vi "VI Tree.vi"   [LabVIEW 2009, in "Keysight XSAn.lvlib"]
doc: "The VI Tree displays all the user-callable VIs of the instrument driver in an organized table."
uses:
  <instrlib>/Keysight XSAn/Keysight XSAn.lvlib
panel:
  # "XSAn"
  # "1.2.3"
  # "SEE DIAGRAM\nFOR VI Tree"
  # "© Keysight Technologies 2015-2021"
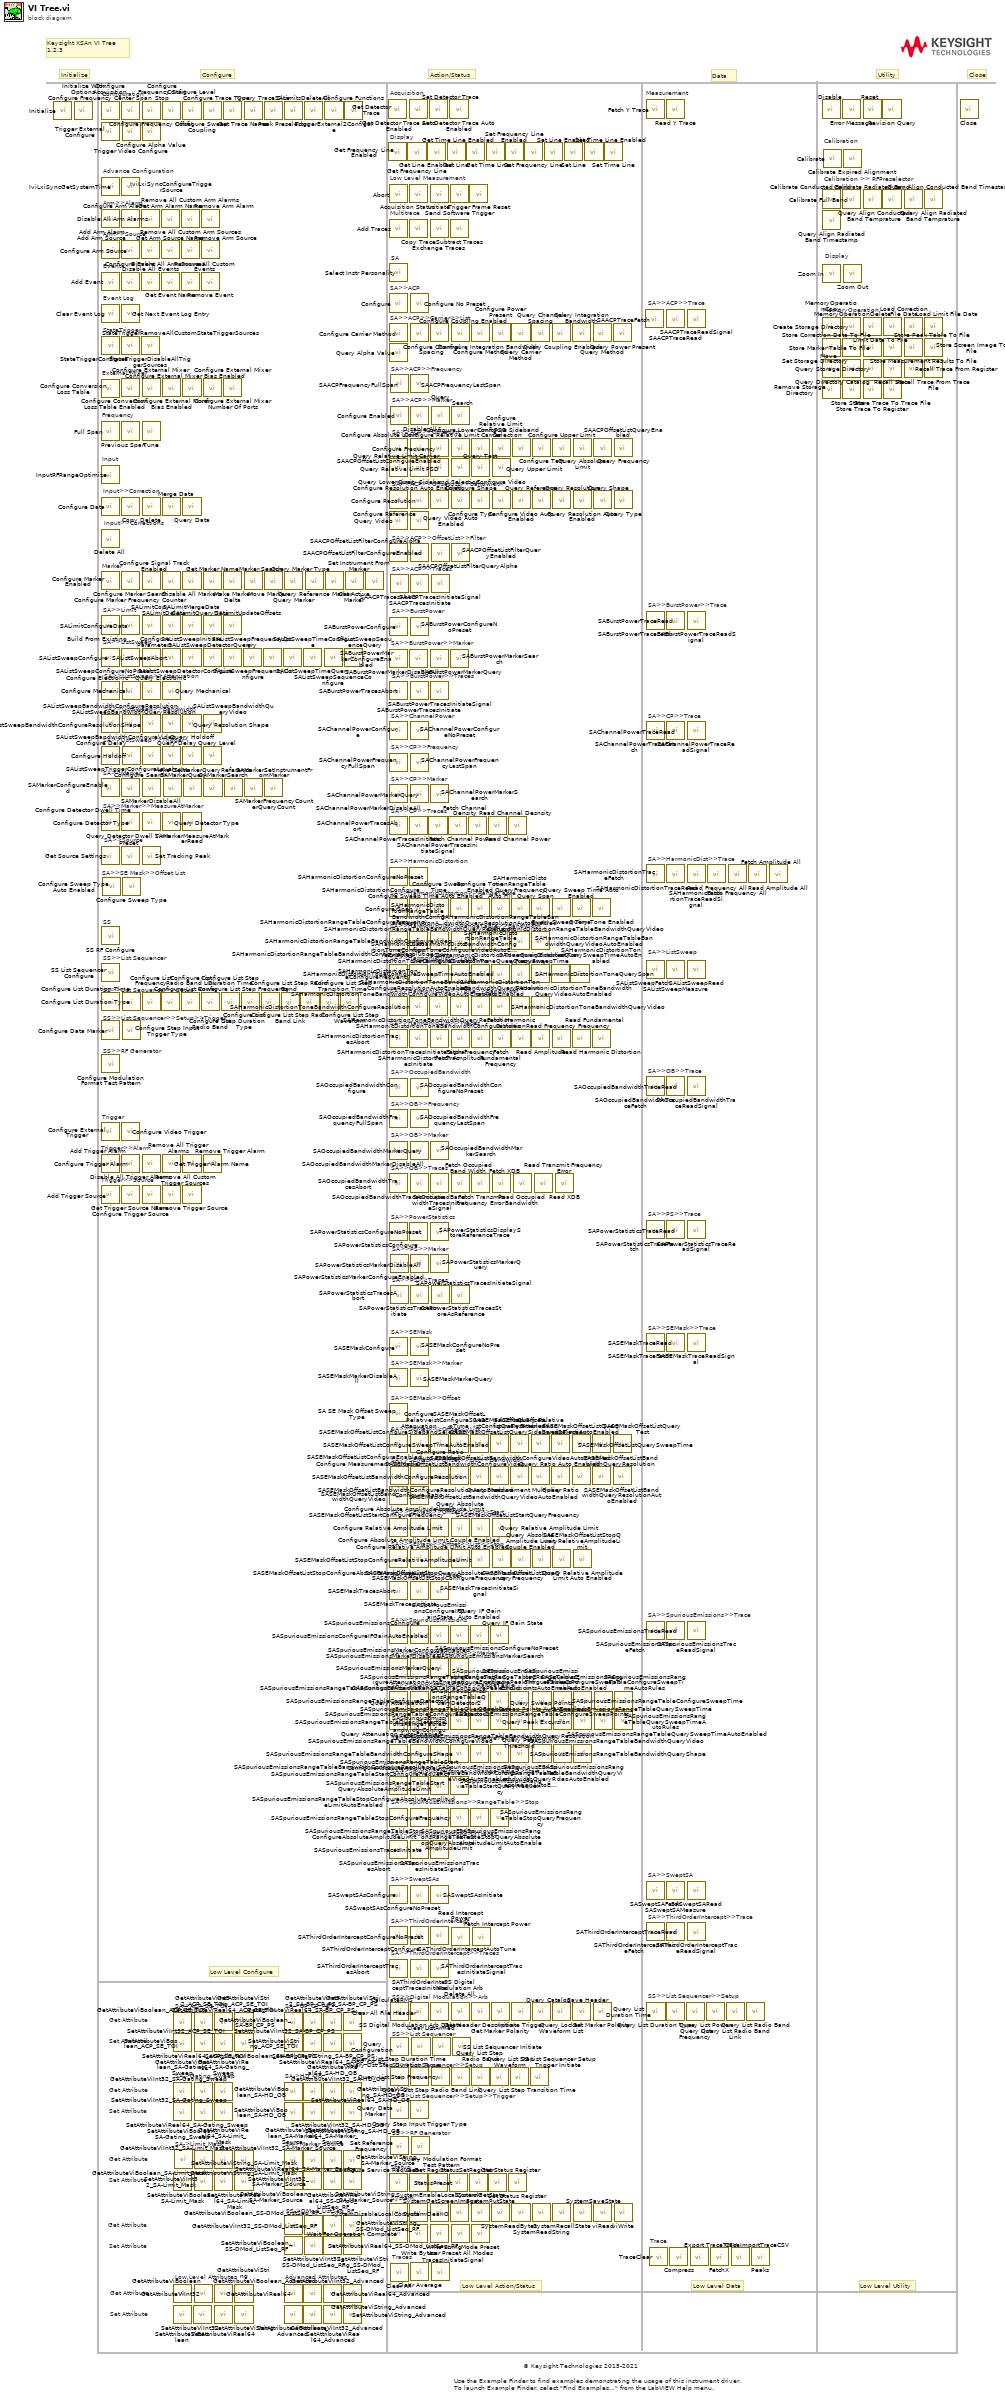
[diagram p0: block diagram]
diagram:
  # "Display"
  # "SA>>SE Mask>>Offset List"
  # "SS>>List Sequencer>>Setup"
  # "SS>>RF Generator"
  # "SS>>List Sequencer>>Setup>>Trigger"
  # "SS>>List Sequencer>>Setup"
  # "SS>>List Sequencer"
  # "SS>>RF Generator"
  # "SS>>List Sequencer>>Setup>>Trigger"
  # "SS>>List Sequencer>>Setup"
  # "SS>>List Sequencer"
  # "SS>>Digital Modulation>>Arb"
  # "SA>>SEMask>>Offset"
  # "SS->DMod_ListSeq_RF"
  # "Set Attribute"
  # "Get Attribute"
  # "SS"
  # "Advance Configuration"
  # "Set Attribute"
  # "Get Attribute"
  # "Set Attribute"
  # "Get Attribute"
  # "Set Attribute"
  # "Get Attribute"
  # "SA->HD_OB"
  # "SA->Marker_Source"
  # "SA->Limit_Mask"
  # "SA->Gating_Sweep"
  # "SA->BP_CP_PS"
  # "SA->ACP_SE_TOI"
  # "Advanced Attributes"
  # "Low Level Attributes"
  # "Trace"
  # "SA>>ListSweep"
  # "SA>>SweptSAs"
  # "SA>>SpuriousEmissions>>RangeTable>>Stop"
  # "SA>>SpuriousEmissions>>RangeTable>>Start"
  # "SA>>SpuriousEmissions>>RangeTable>>Bandwidth"
  # "SA>>SpuriousEmissions>>RangeTable"
  # "SA>>SpuriousEmissions"
  # "SA>>SEMask>>Offset>>List>>Stop"
  # "SA>>SEMask>>Offset>>List>>Start"
  # "SA>>SEMask>>Offset>>List>>Bandwidth"
  # "SA>>SEMask>>Offset>>List"
  # "SA>>Marker>>MeasureAtMarker"
  # "SA>>Marker"
  # "SA>>ListSweep>>Trigger"
  # "SA>>ListSweep>>Bandwidth"
  # "SA>>ListSweep>>Attenuation"
  # "SA>>ListSweep"
  # "SA>>HarmonicDist>>Tone>>Bandwidth"
  # "SA>>HarmonicDist>>Tone"
  # "SA>>HarmonicDist>>RangeTable>>Bandwidth"
  # "SA>>HarmonicDistortion>>RangeTable"
  # "SA>>ACP>>OffsetList>>Filter"
  # "SA>>ACP>>OffsetList>>Bandwidth"
  # "SA>>ACP>>OffsetList"
  # "Set Attribute"
  # "Get Attribute"
  # "© Keysight Technologies 2015-2021"
  # "Low Level Utility"
  # "Low Level Configure"
  # "Low Level Action/Status"
  # "Low Level Data"
  # "Action/Status"
  # "Keysight XSAn VI Tree\n1.2.3"
  # "Close"
  # "Utility"
  # "Data"
  # "Configure"
  # "Initialize"
  # "Use the Example Finder to find examples demonstrating the usage of this instrument driver.\nTo launch Example Finder, select \"Find Examples...\" from the LabVIEW Help menu."
  # "Traces"
  # "System"
  # "Status"
  # "StateTrigger"
  # "SA>>ThirdOrderIntercept>>Traces"
  # "SA>>ThirdOrderIntercept>>Trace"
  # "SA>>ThirdOrderIntercept"
  # "SA>>SweptSA"
  # "SA>>SpuriousEmissions>>Traces"
  # "SA>>SpuriousEmissions>>Trace"
  # "SA>>SpuriousEmissions>>Marker"
  # "SA>>Source"
  # "SA>>SEMask>>Traces"
  # "SA>>SEMask>>Trace"
  # "SA>>SEMask>>Marker"
  # "SA>>SEMask"
  # "SA>>PS>>Traces"
  # "SA>>PS>>Trace"
  # "SA>>PS>>Marker"
  # "SA>>PowerStatistics"
  # "SA>>OB>>Traces"
  # "SA>>OB>>Trace"
  # "SA>>OB>>Marker"
  # "SA>>OB>>Frequency"
  # "SA>>OccupiedBandwidth"
  # "SA>>Limit"
  # "SA>>HarmonicDist>>Traces"
  # "SA>>HarmonicDist>>Trace"
  # "SA>>HarmonicDistortion"
  # "SA>>CP>>Traces"
  # "SA>>CP>>Trace"
  # "SA>>CP>>Marker"
  # "SA>>CP>>Frequency"
  # "SA>>ChannelPower"
  # "SA>>BurstPower>>Traces"
  # "SA>>BurstPower>>Trace"
  # "SA>>BurstPower>>Marker"
  # "SA>>BurstPower"
  # "SA>>ACP>>Traces"
  # "SA>>ACP>>Trace"
  # "SA>>ACP>>Marker"
  # "SA>>ACP>>Frequency"
  # "SA>>ACP>>Carrier>>List"
  # "SA>>ACP"
  # "SA"
  # "MemoryOperation"
  # "Low Level Measurement"
  # "Measurement"
  # "Input>>Corrections"
  # "Input>>Correction"
  # "Input"
  # "Frequency"
  # "Event Log"
  # "Display"
  # "Trigger>>Source"
  # "Trigger>>Alarm"
  # "Trigger"
  # "Multitrace"
  # "Marker"
  # "External Mixer"
  # "Event"
  # "Arm>>Source"
  # "Arm>>Alarm"
  # "Configuration"
  # "Calibration >> RFPreselector"
  # "Calibration"
  # "Acquisition"
  n1 = call <instrlib>:"Initialize.vi"() -> ()  [unwired: 10 in, 2 out]
  n2 = call <instrlib>:"Initialize With Options.vi"() -> ()  [unwired: 10 in, 2 out]
  n3 = call <instrlib>:"Configure Acquisition.vi"() -> ()  [unwired: 10 in, 2 out]
  n4 = call <instrlib>:"Trigger External Configure.vi"() -> ()  [unwired: 10 in, 2 out]
  n5 = call <instrlib>:"Configure Conversion Loss Table.vi"() -> ()  [unwired: 10 in, 2 out]
  n6 = call <instrlib>:"Full Span.vi"() -> ()  [unwired: 10 in, 2 out]
  n7 = call <instrlib>:"InputRFRangeOptimize.vi"() -> ()  [unwired: 10 in, 2 out]
  n8 = call <instrlib>:"Configure Data.vi"() -> ()  [unwired: 10 in, 2 out]
  n9 = call <instrlib>:"Delete All.vi"() -> ()  [unwired: 10 in, 2 out]
  n10 = call <instrlib>:"Configure Marker Enabled.vi"() -> ()  [unwired: 10 in, 2 out]
  n11 = call <instrlib>:"Build From Existing.vi"() -> ()  [unwired: 10 in, 2 out]
  n12 = call <instrlib>:"SAListSweepConfigure.vi"() -> ()  [unwired: 10 in, 2 out]
  n13 = call <instrlib>:"SAMarkerConfigureEnabled.vi"() -> ()  [unwired: 10 in, 2 out]
  n14 = call <instrlib>:"Configure Detector Dwell Time.vi"() -> ()  [unwired: 10 in, 2 out]
  n15 = call <instrlib>:"Get Source Settings.vi"() -> ()  [unwired: 8 in, 4 out]
  n16 = call <instrlib>:"Configure External Trigger.vi"() -> ()  [unwired: 10 in, 2 out]
  n17 = call <instrlib>:"Add Trigger Alarm.vi"() -> ()  [unwired: 10 in, 2 out]
  n18 = call <instrlib>:"Add Trigger Source.vi"() -> ()  [unwired: 10 in, 2 out]
  n19 = call <instrlib>:"IviLxiSyncGetSystemTime.vi"() -> ()  [unwired: 8 in, 4 out]
  n20 = call <instrlib>:"Add Arm Alarm.vi"() -> ()  [unwired: 10 in, 2 out]
  n21 = call <instrlib>:"Add Arm Source.vi"() -> ()  [unwired: 10 in, 2 out]
  n22 = call <instrlib>:"Add Event.vi"() -> ()  [unwired: 10 in, 2 out]
  n23 = call <instrlib>:"Clear Event Log.vi"() -> ()  [unwired: 10 in, 2 out]
  n24 = call <instrlib>:"StateTriggerConfigure.vi"() -> ()  [unwired: 10 in, 2 out]
  n25 = call <instrlib>:"Configure Electronic.vi"() -> ()  [unwired: 10 in, 2 out]
  n26 = call <instrlib>:"SAListSweepBandwidthConfigureResolution.vi"() -> ()  [unwired: 10 in, 2 out]
  n27 = call <instrlib>:"Configure Delay.vi"() -> ()  [unwired: 10 in, 2 out]
  n28 = call <instrlib>:"SS RF Configure.vi"() -> ()  [unwired: 10 in, 2 out]
  n29 = call <instrlib>:"SS List Sequencer Configure.vi"() -> ()  [unwired: 14 in, 2 out]
  n30 = call <instrlib>:"Configure List Duration Time.vi"() -> ()  [unwired: 10 in, 2 out]
  n31 = call <instrlib>:"Configure Data Marker.vi"() -> ()  [unwired: 10 in, 2 out]
  n32 = call <instrlib>:"Configure Modulation Format Test Pattern.vi"() -> ()  [unwired: 10 in, 2 out]
  n33 = call <instrlib>:"Configure Sweep Type Auto Enabled.vi"() -> ()  [unwired: 10 in, 2 out]
  n34 = call <instrlib>:"Configure Frequency Center Span.vi"() -> ()  [unwired: 10 in, 2 out]
  n35 = call <instrlib>:"IviLxiSyncConfigureTriggerSource.vi"() -> ()  [unwired: 10 in, 2 out]
  n36 = call <instrlib>:"Configure Arm Alarm.vi"() -> ()  [unwired: 10 in, 2 out]
  n37 = call <instrlib>:"Configure Arm Source.vi"() -> ()  [unwired: 10 in, 2 out]
  n38 = call <instrlib>:"Configure Event.vi"() -> ()  [unwired: 10 in, 2 out]
  n39 = call <instrlib>:"Get Next Event Log Entry.vi"() -> ()  [unwired: 9 in, 3 out]
  n40 = call <instrlib>:"StateTriggerRemoveAllCustomStateTriggerSources.vi"() -> ()  [unwired: 10 in, 2 out]
  n41 = call <instrlib>:"Configure Conversion Loss Table Enabled.vi"() -> ()  [unwired: 10 in, 2 out]
  n42 = call <instrlib>:"Previous Span.vi"() -> ()  [unwired: 10 in, 2 out]
  n43 = call <instrlib>:"Copy.vi"() -> ()  [unwired: 10 in, 2 out]
  n44 = call <instrlib>:"Configure Marker Frequency Counter.vi"() -> ()  [unwired: 10 in, 2 out]
  n45 = call <instrlib>:"SALimitConfigureData.vi"() -> ()  [unwired: 10 in, 2 out]
  n46 = call <instrlib>:"SAListSweepConfigureNoPreset.vi"() -> ()  [unwired: 10 in, 2 out]
  n47 = call <instrlib>:"Configure Search.vi"() -> ()  [unwired: 10 in, 2 out]
  n48 = call <instrlib>:"Configure Detector Type.vi"() -> ()  [unwired: 10 in, 2 out]
  n49 = call <instrlib>:"Preset.vi"() -> ()  [unwired: 10 in, 2 out]
  n50 = call <instrlib>:"Configure Video Trigger.vi"() -> ()  [unwired: 10 in, 2 out]
  n51 = call <instrlib>:"Configure Trigger Alarm.vi"() -> ()  [unwired: 10 in, 2 out]
  n52 = call <instrlib>:"Configure Trigger Source.vi"() -> ()  [unwired: 10 in, 2 out]
  n53 = call <instrlib>:"Trigger Video Configure.vi"() -> ()  [unwired: 10 in, 2 out]
  n54 = call <instrlib>:"Configure Mechanical.vi"() -> ()  [unwired: 10 in, 2 out]
  n55 = call <instrlib>:"SAListSweepBandwidthConfigureResolutionShape.vi"() -> ()  [unwired: 10 in, 2 out]
  n56 = call <instrlib>:"Configure Holdoff.vi"() -> ()  [unwired: 10 in, 2 out]
  n57 = call <instrlib>:"Configure List Duration Type.vi"() -> ()  [unwired: 10 in, 2 out]
  n58 = call <instrlib>:"Configure Step Input Trigger Type.vi"() -> ()  [unwired: 10 in, 2 out]
  n59 = call <instrlib>:"Configure Sweep Type.vi"() -> ()  [unwired: 10 in, 2 out]
  n60 = call <instrlib>:"Disable All Arm Alarms.vi"() -> ()  [unwired: 10 in, 2 out]
  n61 = call <instrlib>:"Disable All Arm Sources.vi"() -> ()  [unwired: 10 in, 2 out]
  n62 = call <instrlib>:"Disable All Events.vi"() -> ()  [unwired: 10 in, 2 out]
  n63 = call <instrlib>:"StateTriggerDisableAllTriggerSources.vi"() -> ()  [unwired: 10 in, 2 out]
  n64 = call <instrlib>:"Configure Frequency Offset.vi"() -> ()  [unwired: 10 in, 2 out]
  n65 = call <instrlib>:"Configure Alpha Value.vi"() -> ()  [unwired: 10 in, 2 out]
  n66 = call <instrlib>:"Configure External Mixer.vi"() -> ()  [unwired: 10 in, 2 out]
  n67 = call <instrlib>:"Tune.vi"() -> ()  [unwired: 10 in, 2 out]
  n68 = call <instrlib>:"Delete.vi"() -> ()  [unwired: 10 in, 2 out]
  n69 = call <instrlib>:"Configure Marker Search.vi"() -> ()  [unwired: 10 in, 2 out]
  n70 = call <instrlib>:"SALimitCopy.vi"() -> ()  [unwired: 10 in, 2 out]
  n71 = call <instrlib>:"Configure Parameters.vi"() -> ()  [unwired: 14 in, 2 out]
  n72 = call <instrlib>:"Query Electronic.vi"() -> ()  [unwired: 8 in, 4 out]
  n73 = call <instrlib>:"Query Detector Dwell Time.vi"() -> ()  [unwired: 9 in, 3 out]
  n74 = call <instrlib>:"Set Tracking Peak.vi"() -> ()  [unwired: 10 in, 2 out]
  n75 = call <instrlib>:"Configure List Frequency.vi"() -> ()  [unwired: 10 in, 2 out]
  n76 = call <instrlib>:"Disable All Trigger Alarms.vi"() -> ()  [unwired: 10 in, 2 out]
  n77 = call <instrlib>:"Get Trigger Source Name.vi"() -> ()  [unwired: 9 in, 3 out]
  n78 = call <instrlib>:"SAListSweepBandwidthConfigureVideo.vi"() -> ()  [unwired: 10 in, 2 out]
  n79 = call <instrlib>:"SAListSweepTriggerConfigureLevel.vi"() -> ()  [unwired: 10 in, 2 out]
  n80 = call <instrlib>:"SAMarkerDisableAll.vi"() -> ()  [unwired: 10 in, 2 out]
  n81 = call <instrlib>:"Get Arm Alarm Name.vi"() -> ()  [unwired: 9 in, 3 out]
  n82 = call <instrlib>:"Get Arm Source Name.vi"() -> ()  [unwired: 9 in, 3 out]
  n83 = call <instrlib>:"Get Event Name.vi"() -> ()  [unwired: 9 in, 3 out]
  n84 = call <instrlib>:"Configure List Power.vi"() -> ()  [unwired: 10 in, 2 out]
  n85 = call <instrlib>:"Configure Frequency Start Stop.vi"() -> ()  [unwired: 10 in, 2 out]
  n86 = call <instrlib>:"Configure External Mixer Bias.vi"() -> ()  [unwired: 10 in, 2 out]
  n87 = call <instrlib>:"Merge Data.vi"() -> ()  [unwired: 10 in, 2 out]
  n88 = call <instrlib>:"Configure Signal Track Enabled.vi"() -> ()  [unwired: 10 in, 2 out]
  n89 = call <instrlib>:"SALimitDelete.vi"() -> ()  [unwired: 10 in, 2 out]
  n90 = call <instrlib>:"SAListSweepAbort.vi"() -> ()  [unwired: 10 in, 2 out]
  n91 = call <instrlib>:"Query Mechanical.vi"() -> ()  [unwired: 8 in, 4 out]
  n92 = call <instrlib>:"SAListSweepBandwidthQueryResolution.vi"() -> ()  [unwired: 8 in, 4 out]
  n93 = call <instrlib>:"Query Delay.vi"() -> ()  [unwired: 8 in, 4 out]
  n94 = call <instrlib>:"Query Detector Type.vi"() -> ()  [unwired: 9 in, 3 out]
  n95 = call <instrlib>:"Get Trigger Alarm Name.vi"() -> ()  [unwired: 9 in, 3 out]
  n96 = call <instrlib>:"Remove All Custom Trigger Sources.vi"() -> ()  [unwired: 10 in, 2 out]
  n97 = call <instrlib>:"Make Delta.vi"() -> ()  [unwired: 10 in, 2 out]
  n98 = call <instrlib>:"GetAttributeViBoolean_ACP_SE_TOI.vi"() -> ()  [unwired: 9 in, 3 out]
  n99 = call <instrlib>:"SetAttributeViBoolean_ACP_SE_TOI.vi"() -> ()  [unwired: 10 in, 2 out]
  n100 = call <instrlib>:"GetAttributeViBoolean_SA-Gating_Sweep.vi"() -> ()  [unwired: 9 in, 3 out]
  n101 = call <instrlib>:"SetAttributeViBoolean_SA-Gating_Sweep.vi"() -> ()  [unwired: 10 in, 2 out]
  n102 = call <instrlib>:"SetAttributeViBoolean_SA-Limit_Mask.vi"() -> ()  [unwired: 10 in, 2 out]
  n103 = call <instrlib>:"GetAttributeViBoolean.vi"() -> ()  [unwired: 9 in, 3 out]
  n104 = call <instrlib>:"SetAttributeViBoolean.vi"() -> ()  [unwired: 10 in, 2 out]
  n105 = call <instrlib>:"GetAttributeViBoolean_SA-Limit_Mask.vi"() -> ()  [unwired: 9 in, 3 out]
  n106 = call <instrlib>:"Remove All Custom Arm Alarms.vi"() -> ()  [unwired: 10 in, 2 out]
  n107 = call <instrlib>:"Remove All Custom Arm Sources.vi"() -> ()  [unwired: 10 in, 2 out]
  n108 = call <instrlib>:"Remove All Custom Events.vi"() -> ()  [unwired: 10 in, 2 out]
  n109 = call <instrlib>:"Configure List Radio Band Link.vi"() -> ()  [unwired: 10 in, 2 out]
  n110 = call <instrlib>:"Configure Level.vi"() -> ()  [unwired: 10 in, 2 out]
  n111 = call <instrlib>:"Configure External Mixer Bias Enabled.vi"() -> ()  [unwired: 10 in, 2 out]
  n112 = call <instrlib>:"Query Data.vi"() -> ()  [unwired: 8 in, 4 out]
  n113 = call <instrlib>:"Disable All Markers.vi"() -> ()  [unwired: 10 in, 2 out]
  n114 = call <instrlib>:"SALimitMergeData.vi"() -> ()  [unwired: 10 in, 2 out]
  n115 = call <instrlib>:"SAListSweepInitiate.vi"() -> ()  [unwired: 10 in, 2 out]
  n116 = call <instrlib>:"Query Resolution Shape.vi"() -> ()  [unwired: 8 in, 4 out]
  n117 = call <instrlib>:"Query Holdoff.vi"() -> ()  [unwired: 8 in, 4 out]
  n118 = call <instrlib>:"SAMarkerMeasureAtMarkerRead.vi"() -> ()  [unwired: 8 in, 4 out]
  n119 = call <instrlib>:"Remove All Trigger Alarms.vi"() -> ()  [unwired: 10 in, 2 out]
  n120 = call <instrlib>:"Remove Trigger Source.vi"() -> ()  [unwired: 10 in, 2 out]
  n121 = call <instrlib>:"SAMarkerQuery.vi"() -> ()  [unwired: 8 in, 4 out]
  n122 = call <instrlib>:"SetAttributeViInt32.vi"() -> ()  [unwired: 10 in, 2 out]
  n123 = call <instrlib>:"GetAttributeViInt32_ACP_SE_TOI.vi"() -> ()  [unwired: 9 in, 3 out]
  n124 = call <instrlib>:"SetAttributeViInt32_ACP_SE_TOI.vi"() -> ()  [unwired: 10 in, 2 out]
  n125 = call <instrlib>:"GetAttributeViInt32_SA-Gating_Sweep.vi"() -> ()  [unwired: 9 in, 3 out]
  n126 = call <instrlib>:"SetAttributeViInt32_SA-Gating_Sweep.vi"() -> ()  [unwired: 10 in, 2 out]
  n127 = call <instrlib>:"GetAttributeViInt32_SA-Limit_Mask.vi"() -> ()  [unwired: 9 in, 3 out]
  n128 = call <instrlib>:"SetAttributeViInt32_SA-Limit_Mask.vi"() -> ()  [unwired: 10 in, 2 out]
  n129 = call <instrlib>:"GetAttributeViInt32.vi"() -> ()  [unwired: 9 in, 3 out]
  n130 = call <instrlib>:"Remove Arm Alarm.vi"() -> ()  [unwired: 10 in, 2 out]
  n131 = call <instrlib>:"Remove Arm Source.vi"() -> ()  [unwired: 10 in, 2 out]
  n132 = call <instrlib>:"Remove Event.vi"() -> ()  [unwired: 10 in, 2 out]
  n133 = call <instrlib>:"Configure List Radio Band.vi"() -> ()  [unwired: 10 in, 2 out]
  n134 = call <instrlib>:"Configure Sweep Coupling.vi"() -> ()  [unwired: 10 in, 2 out]
  n135 = call <instrlib>:"Configure External Mixer Enabled.vi"() -> ()  [unwired: 10 in, 2 out]
  n136 = call <instrlib>:"Get Marker Name.vi"() -> ()  [unwired: 9 in, 3 out]
  n137 = call <instrlib>:"SALimitQueryData.vi"() -> ()  [unwired: 8 in, 4 out]
  n138 = call <instrlib>:"SAListSweepDetectorConfigure.vi"() -> ()  [unwired: 10 in, 2 out]
  n139 = call <instrlib>:"SAListSweepBandwidthQueryVideo.vi"() -> ()  [unwired: 8 in, 4 out]
  n140 = call <instrlib>:"Query Level.vi"() -> ()  [unwired: 8 in, 4 out]
  n141 = call <instrlib>:"Remove Trigger Alarm.vi"() -> ()  [unwired: 10 in, 2 out]
  n142 = call <instrlib>:"SAMarkerQueryReference.vi"() -> ()  [unwired: 8 in, 4 out]
  n143 = call <instrlib>:"GetAttributeViReal64_ACP_SE_TOI.vi"() -> ()  [unwired: 9 in, 3 out]
  n144 = call <instrlib>:"SetAttributeViReal64_ACP_SE_TOI.vi"() -> ()  [unwired: 10 in, 2 out]
  n145 = call <instrlib>:"GetAttributeViReal64_SA-Gating_Sweep.vi"() -> ()  [unwired: 9 in, 3 out]
  n146 = call <instrlib>:"SetAttributeViReal64_SA-Gating_Sweep.vi"() -> ()  [unwired: 10 in, 2 out]
  n147 = call <instrlib>:"GetAttributeViReal64_SA-Limit_Mask.vi"() -> ()  [unwired: 9 in, 3 out]
  n148 = call <instrlib>:"SetAttributeViReal64_SA-Limit_Mask.vi"() -> ()  [unwired: 10 in, 2 out]
  n149 = call <instrlib>:"GetAttributeViReal64.vi"() -> ()  [unwired: 9 in, 3 out]
  n150 = call <instrlib>:"SetAttributeViReal64.vi"() -> ()  [unwired: 10 in, 2 out]
  n151 = call <instrlib>:"Configure List Step Duration Time.vi"() -> ()  [unwired: 10 in, 2 out]
  n152 = call <instrlib>:"Configure Trace Type.vi"() -> ()  [unwired: 10 in, 2 out]
  n153 = call <instrlib>:"Configure External Mixer Number Of Ports.vi"() -> ()  [unwired: 10 in, 2 out]
  n154 = call <instrlib>:"Make Marker Delta.vi"() -> ()  [unwired: 10 in, 2 out]
  n155 = call <instrlib>:"SALimitUpdateOffsets.vi"() -> ()  [unwired: 10 in, 2 out]
  n156 = call <instrlib>:"SAListSweepDetectorQuery.vi"() -> ()  [unwired: 8 in, 4 out]
  n157 = call <instrlib>:"SAMarkerSearch.vi"() -> ()  [unwired: 10 in, 2 out]
  n158 = call <instrlib>:"GetAttributeViString_ACP_SE_TOI.vi"() -> ()  [unwired: 9 in, 3 out]
  n159 = call <instrlib>:"SetAttributeViString_ACP_SE_TOI.vi"() -> ()  [unwired: 10 in, 2 out]
  n160 = call <instrlib>:"GetAttributeViString_SA-Limit_Mask.vi"() -> ()  [unwired: 9 in, 3 out]
  n161 = call <instrlib>:"SetAttributeViString_SA-Limit_Mask.vi"() -> ()  [unwired: 10 in, 2 out]
  n162 = call <instrlib>:"GetAttributeViString.vi"() -> ()  [unwired: 9 in, 3 out]
  n163 = call <instrlib>:"SetAttributeViString.vi"() -> ()  [unwired: 10 in, 2 out]
  n164 = call <instrlib>:"Configure List Step Duration Type.vi"() -> ()  [unwired: 10 in, 2 out]
  n165 = call <instrlib>:"SAListSweepFrequencyConfigure.vi"() -> ()  [unwired: 10 in, 2 out]
  n166 = call <instrlib>:"Get Trace Name.vi"() -> ()  [unwired: 9 in, 3 out]
  n167 = call <instrlib>:"Marker Search.vi"() -> ()  [unwired: 10 in, 2 out]
  n168 = call <instrlib>:"SAMarkerSetInstrumentFromMarker.vi"() -> ()  [unwired: 10 in, 2 out]
  n169 = call <instrlib>:"Configure List Step Frequency.vi"() -> ()  [unwired: 10 in, 2 out]
  n170 = call <instrlib>:"SAListSweepFrequencyQuery.vi"() -> ()  [unwired: 8 in, 4 out]
  n171 = call <instrlib>:"Query Trace Size.vi"() -> ()  [unwired: 9 in, 3 out]
  n172 = call <instrlib>:"Move Marker.vi"() -> ()  [unwired: 10 in, 2 out]
  n173 = call <instrlib>:"SAMarkerFrequencyCounterQueryCount.vi"() -> ()  [unwired: 9 in, 3 out]
  n174 = call <instrlib>:"Configure List Step Radio Band Link.vi"() -> ()  [unwired: 10 in, 2 out]
  n175 = call <instrlib>:"SAListSweepTimeConfigure.vi"() -> ()  [unwired: 10 in, 2 out]
  n176 = call <instrlib>:"GetAttributeViBoolean_SA-BP_CP_PS.vi"() -> ()  [unwired: 9 in, 3 out]
  n177 = call <instrlib>:"SetAttributeViBoolean_SA-BP_CP_PS.vi"() -> ()  [unwired: 10 in, 2 out]
  n178 = call <instrlib>:"GetAttributeViBoolean_SA-HD_OB.vi"() -> ()  [unwired: 9 in, 3 out]
  n179 = call <instrlib>:"SetAttributeViBoolean_SA-HD_OB.vi"() -> ()  [unwired: 10 in, 2 out]
  n180 = call <instrlib>:"GetAttributeViBoolean_SA-Marker_Source.vi"() -> ()  [unwired: 9 in, 3 out]
  n181 = call <instrlib>:"SetAttributeViBoolean_SA-Marker_Source.vi"() -> ()  [unwired: 10 in, 2 out]
  n182 = call <instrlib>:"GetAttributeViBoolean_Advanced.vi"() -> ()  [unwired: 9 in, 3 out]
  n183 = call <instrlib>:"SetAttributeViBoolean_Advanced.vi"() -> ()  [unwired: 10 in, 2 out]
  n184 = call <instrlib>:"Peak Preselector.vi"() -> ()  [unwired: 10 in, 2 out]
  n185 = call <instrlib>:"Query Marker.vi"() -> ()  [unwired: 8 in, 4 out]
  n186 = call <instrlib>:"GetAttributeViBoolean_SS-DMod_ListSeq_RF.vi"() -> ()  [unwired: 9 in, 3 out]
  n187 = call <instrlib>:"SetAttributeViBoolean_SS-DMod_ListSeq_RF.vi"() -> ()  [unwired: 10 in, 2 out]
  n188 = call <instrlib>:"Configure List Step Radio Band.vi"() -> ()  [unwired: 10 in, 2 out]
  n189 = call <instrlib>:"SAListSweepTimeQuery.vi"() -> ()  [unwired: 8 in, 4 out]
  n190 = call <instrlib>:"GetAttributeViInt32_SA-BP_CP_PS.vi"() -> ()  [unwired: 9 in, 3 out]
  n191 = call <instrlib>:"SetAttributeViInt32_SA-BP_CP_PS.vi"() -> ()  [unwired: 10 in, 2 out]
  n192 = call <instrlib>:"GetAttributeViInt32_SA-HD_OB.vi"() -> ()  [unwired: 9 in, 3 out]
  n193 = call <instrlib>:"SetAttributeViInt32_SA-HD_OB.vi"() -> ()  [unwired: 10 in, 2 out]
  n194 = call <instrlib>:"GetAttributeViInt32_SA-Marker_Source.vi"() -> ()  [unwired: 9 in, 3 out]
  n195 = call <instrlib>:"SetAttributeViInt32_SA-Marker_Source.vi"() -> ()  [unwired: 10 in, 2 out]
  n196 = call <instrlib>:"GetAttributeViInt32_Advanced.vi"() -> ()  [unwired: 9 in, 3 out]
  n197 = call <instrlib>:"SetAttributeViInt32_Advanced.vi"() -> ()  [unwired: 10 in, 2 out]
  n198 = call <instrlib>:"SALimitsDeleteAll.vi"() -> ()  [unwired: 10 in, 2 out]
  n199 = call <instrlib>:"GetAttributeViInt32_SS-DMod_ListSeq_RF.vi"() -> ()  [unwired: 9 in, 3 out]
  n200 = call <instrlib>:"SetAttributeViInt32_SS-DMod_ListSeq_RF.vi"() -> ()  [unwired: 10 in, 2 out]
  n201 = call <instrlib>:"Query Marker Type.vi"() -> ()  [unwired: 9 in, 3 out]
  n202 = call <instrlib>:"Configure List Step Transition Time.vi"() -> ()  [unwired: 10 in, 2 out]
  n203 = call <instrlib>:"GetAttributeViReal64_SA-BP_CP_PS.vi"() -> ()  [unwired: 9 in, 3 out]
  n204 = call <instrlib>:"SetAttributeViReal64_SA-BP_CP_PS.vi"() -> ()  [unwired: 10 in, 2 out]
  n205 = call <instrlib>:"GetAttributeViReal64_SA-HD_OB.vi"() -> ()  [unwired: 9 in, 3 out]
  n206 = call <instrlib>:"SetAttributeViReal64_SA-HD_OB.vi"() -> ()  [unwired: 10 in, 2 out]
  n207 = call <instrlib>:"GetAttributeViReal64_SA-Marker_Source.vi"() -> ()  [unwired: 9 in, 3 out]
  n208 = call <instrlib>:"SetAttributeViReal64_SA-Marker_Source.vi"() -> ()  [unwired: 10 in, 2 out]
  n209 = call <instrlib>:"GetAttributeViReal64_SS-DMod_ListSeq_RF.vi"() -> ()  [unwired: 9 in, 3 out]
  n210 = call <instrlib>:"SetAttributeViReal64_SS-DMod_ListSeq_RF.vi"() -> ()  [unwired: 9 in, 2 out]
  n211 = call <instrlib>:"GetAttributeViReal64_Advanced.vi"() -> ()  [unwired: 9 in, 3 out]
  n212 = call <instrlib>:"SetAttributeViReal64_Advanced.vi"() -> ()  [unwired: 10 in, 2 out]
  n213 = call <instrlib>:"SAListSweepSequenceConfigure.vi"() -> ()  [unwired: 10 in, 2 out]
  n214 = call <instrlib>:"TriggerExternal2Configure.vi"() -> ()  [unwired: 10 in, 2 out]
  n215 = call <instrlib>:"Query Reference Marker.vi"() -> ()  [unwired: 8 in, 4 out]
  n216 = call <instrlib>:"Configure List Step Waveform.vi"() -> ()  [unwired: 10 in, 2 out]
  n217 = call <instrlib>:"GetAttributeViString_SA-BP_CP_PS.vi"() -> ()  [unwired: 9 in, 3 out]
  n218 = call <instrlib>:"SetAttributeViString_SA-BP_CP_PS.vi"() -> ()  [unwired: 10 in, 2 out]
  n219 = call <instrlib>:"GetAttributeViString_SA-HD_OB.vi"() -> ()  [unwired: 9 in, 3 out]
  n220 = call <instrlib>:"SetAttributeViString_SA-HD_OB.vi"() -> ()  [unwired: 10 in, 2 out]
  n221 = call <instrlib>:"GetAttributeViString_SA-Marker_Source.vi"() -> ()  [unwired: 9 in, 3 out]
  n222 = call <instrlib>:"SetAttributeViString_SA-Marker_Source.vi"() -> ()  [unwired: 10 in, 2 out]
  n223 = call <instrlib>:"GetAttributeViString_SS-DMod_ListSeq_RF.vi"() -> ()  [unwired: 9 in, 3 out]
  n224 = call <instrlib>:"SetAttributeViString_SS-DMod_ListSeq_RF.vi"() -> ()  [unwired: 10 in, 2 out]
  n225 = call <instrlib>:"GetAttributeViString_Advanced.vi"() -> ()  [unwired: 9 in, 3 out]
  n226 = call <instrlib>:"SetAttributeViString_Advanced.vi"() -> ()  [unwired: 10 in, 2 out]
  n227 = call <instrlib>:"Configure Functions.vi"() -> ()  [unwired: 14 in, 2 out]
  n228 = call <instrlib>:"SAListSweepSequenceQuery.vi"() -> ()  [unwired: 8 in, 4 out]
  n229 = call <instrlib>:"Set Active Marker.vi"() -> ()  [unwired: 10 in, 2 out]
  n230 = call <instrlib>:"Set Instrument From Marker.vi"() -> ()  [unwired: 10 in, 2 out]
  n231 = call <instrlib>:"Get Detector Trace.vi"() -> ()  [unwired: 9 in, 3 out]
  n232 = call <instrlib>:"Get Frequency Line Enabled.vi"() -> ()  [unwired: 9 in, 3 out]
  n233 = call <instrlib>:"Abort.vi"() -> ()  [unwired: 10 in, 2 out]
  n234 = call <instrlib>:"Add Traces.vi"() -> ()  [unwired: 10 in, 2 out]
  n235 = call <instrlib>:"Select Instr Personality.vi"() -> ()  [unwired: 10 in, 2 out]
  n236 = call <instrlib>:"Configure.vi"() -> ()  [unwired: 10 in, 2 out]
  n237 = call <instrlib>:"Configure Carrier Method.vi"() -> ()  [unwired: 8 in, 3 out]
  n238 = call <instrlib>:"Query Alpha Value.vi"() -> ()  [unwired: 8 in, 4 out]
  n239 = call <instrlib>:"SABurstPowerMarkerConfigureEnabled.vi"() -> ()  [unwired: 10 in, 2 out]
  n240 = call <instrlib>:"SAHarmonicDistortionConfigure.vi"() -> ()  [unwired: 10 in, 2 out]
  n241 = call <instrlib>:"SAHarmonicDistortionRangeTableConfigureFrequency.vi"() -> ()  [unwired: 10 in, 2 out]
  n242 = call <instrlib>:"SAHarmonicDistortionRangeTableBandwidthConfigureResolution.vi"() -> ()  [unwired: 10 in, 2 out]
  n243 = call <instrlib>:"SAHarmonicDistortionToneConfigureEnabled.vi"() -> ()  [unwired: 10 in, 2 out]
  n244 = call <instrlib>:"SAHarmonicDistortionToneBandwidthConfigureResolution.vi"() -> ()  [unwired: 10 in, 2 out]
  n245 = call <instrlib>:"SAHarmonicDistortionTracesAbort.vi"() -> ()  [unwired: 10 in, 2 out]
  n246 = call <instrlib>:"SAPowerStatisticsConfigure.vi"() -> ()  [unwired: 10 in, 2 out]
  n247 = call <instrlib>:"Configure Service Request.vi"() -> ()  [unwired: 10 in, 2 out]
  n248 = call <instrlib>:"SystemClearIO.vi"() -> ()  [unwired: 10 in, 2 out]
  n249 = call <instrlib>:"Wait For Operation Complete.vi"() -> ()  [unwired: 10 in, 2 out]
  n250 = call <instrlib>:"Configure Absolute Limit.vi"() -> ()  [unwired: 10 in, 2 out]
  n251 = call <instrlib>:"Query Lower Limit.vi"() -> ()  [unwired: 8 in, 4 out]
  n252 = call <instrlib>:"Configure Reference.vi"() -> ()  [unwired: 10 in, 2 out]
  n253 = call <instrlib>:"Query Video.vi"() -> ()  [unwired: 8 in, 4 out]
  n254 = call <instrlib>:"SAACPOffsetListFilterConfigureAlpha.vi"() -> ()  [unwired: 10 in, 2 out]
  n255 = call <instrlib>:"SABurstPowerConfigure.vi"() -> ()  [unwired: 10 in, 2 out]
  n256 = call <instrlib>:"SABurstPowerTracesAbort.vi"() -> ()  [unwired: 10 in, 2 out]
  n257 = call <instrlib>:"SAChannelPowerConfigure.vi"() -> ()  [unwired: 10 in, 2 out]
  n258 = call <instrlib>:"SAChannelPowerFrequencyFullSpan.vi"() -> ()  [unwired: 10 in, 2 out]
  n259 = call <instrlib>:"SAChannelPowerMarkerDisableAll.vi"() -> ()  [unwired: 10 in, 2 out]
  n260 = call <instrlib>:"SAChannelPowerTracesAbort.vi"() -> ()  [unwired: 10 in, 2 out]
  n261 = call <instrlib>:"SAOccupiedBandwidthConfigure.vi"() -> ()  [unwired: 10 in, 2 out]
  n262 = call <instrlib>:"SAOccupiedBandwidthFrequencyFullSpan.vi"() -> ()  [unwired: 10 in, 2 out]
  n263 = call <instrlib>:"SAOccupiedBandwidthMarkerDisableAll.vi"() -> ()  [unwired: 10 in, 2 out]
  n264 = call <instrlib>:"SAOccupiedBandwidthTracesAbort.vi"() -> ()  [unwired: 10 in, 2 out]
  n265 = call <instrlib>:"SASEMaskConfigure.vi"() -> ()  [unwired: 10 in, 2 out]
  n266 = call <instrlib>:"SASEMaskMarkerDisableAll.vi"() -> ()  [unwired: 10 in, 2 out]
  n267 = call <instrlib>:"SA SE Mask Offset Sweep Type.vi"() -> ()  [unwired: 8 in, 4 out]
  n268 = call <instrlib>:"SASEMaskOffsetListConfigureEnabled.vi"() -> ()  [unwired: 10 in, 2 out]
  n269 = call <instrlib>:"SASEMaskOffsetListBandwidthQueryVideo.vi"() -> ()  [unwired: 8 in, 4 out]
  n270 = call <instrlib>:"Configure Absolute Amplitude Limit.vi"() -> ()  [unwired: 10 in, 2 out]
  n271 = call <instrlib>:"SASEMaskOffsetListStopConfigureAbsoluteAmplitudeLimit.vi"() -> ()  [unwired: 10 in, 2 out]
  n272 = call <instrlib>:"SASEMaskTracesAbort.vi"() -> ()  [unwired: 10 in, 2 out]
  n273 = call <instrlib>:"SASpuriousEmissionsConfigure.vi"() -> ()  [unwired: 10 in, 2 out]
  n274 = call <instrlib>:"SASpuriousEmissionsMarkerConfigureEnabled.vi"() -> ()  [unwired: 10 in, 2 out]
  n275 = call <instrlib>:"SASpuriousEmissionsRangeTableConfigureAttenuation.vi"() -> ()  [unwired: 10 in, 2 out]
  n276 = call <instrlib>:"Query Attenuation.vi"() -> ()  [unwired: 8 in, 4 out]
  n277 = call <instrlib>:"SASpuriousEmissionsRangeTableBandwidthConfigureResolution.vi"() -> ()  [unwired: 10 in, 2 out]
  n278 = call <instrlib>:"SASpuriousEmissionsRangeTableStartConfigureAbsoluteAmplitudeLimit.vi"() -> ()  [unwired: 10 in, 2 out]
  n279 = call <instrlib>:"SASpuriousEmissionsRangeTableStopConfigureAbsoluteAmplitudeLimit.vi"() -> ()  [unwired: 10 in, 2 out]
  n280 = call <instrlib>:"SASpuriousEmissionsTracesAbort.vi"() -> ()  [unwired: 10 in, 2 out]
  n281 = call <instrlib>:"SASweptSAsConfigure.vi"() -> ()  [unwired: 10 in, 2 out]
  n282 = call <instrlib>:"SAThirdOrderInterceptConfigure.vi"() -> ()  [unwired: 10 in, 2 out]
  n283 = call <instrlib>:"SAThirdOrderInterceptTracesAbort.vi"() -> ()  [unwired: 10 in, 2 out]
  n284 = call <instrlib>:"SAACPFrequencyFullSpan.vi"() -> ()  [unwired: 10 in, 2 out]
  n285 = call <instrlib>:"Configure Enabled.vi"() -> ()  [unwired: 10 in, 2 out]
  n286 = call <instrlib>:"SAACPTracesAbort.vi"() -> ()  [unwired: 10 in, 2 out]
  n287 = call <instrlib>:"SAPowerStatisticsMarkerConfigureEnabled.vi"() -> ()  [unwired: 10 in, 2 out]
  n288 = call <instrlib>:"SAPowerStatisticsTracesAbort.vi"() -> ()  [unwired: 10 in, 2 out]
  n289 = call <instrlib>:"Configure Measurement Multiplier.vi"() -> ()  [unwired: 10 in, 2 out]
  n290 = call <instrlib>:"CalculateRMS.vi"() -> ()  [unwired: 10 in, 2 out]
  n291 = call <instrlib>:"Query Configuration.vi"() -> ()  [unwired: 4 in, 12 out]
  n292 = call <instrlib>:"Query List Step Duration Time.vi"() -> ()  [unwired: 9 in, 3 out]
  n293 = call <instrlib>:"Query Data Marker.vi"() -> ()  [unwired: 9 in, 3 out]
  n294 = call <instrlib>:"Set Reference Frequency.vi"() -> ()  [unwired: 10 in, 2 out]
  n295 = call <instrlib>:"Clear All.vi"() -> ()  [unwired: 10 in, 2 out]
  n296 = call <instrlib>:"Get Frequency Line.vi"() -> ()  [unwired: 9 in, 3 out]
  n297 = call <instrlib>:"Get Detector Trace Auto Enabled.vi"() -> ()  [unwired: 9 in, 3 out]
  n298 = call <instrlib>:"SAChannelPowerTracesInitiate.vi"() -> ()  [unwired: 10 in, 2 out]
  n299 = call <instrlib>:"Clear.vi"() -> ()  [unwired: 10 in, 2 out]
  n300 = call <instrlib>:"Acquisition Status.vi"() -> ()  [unwired: 9 in, 3 out]
  n301 = call <instrlib>:"Copy Trace.vi"() -> ()  [unwired: 10 in, 2 out]
  n302 = call <instrlib>:"SABurstPowerMarkerDisableAll.vi"() -> ()  [unwired: 10 in, 2 out]
  n303 = call <instrlib>:"SAHarmonicDistortionConfigureNoPreset.vi"() -> ()  [unwired: 10 in, 2 out]
  n304 = call <instrlib>:"Configure Span.vi"() -> ()  [unwired: 10 in, 2 out]
  n305 = call <instrlib>:"SAHarmonicDistortionRangeTableBandwidthConfigureResolutionAutoEnabled.vi"() -> ()  [unwired: 10 in, 2 out]
  n306 = call <instrlib>:"SAHarmonicDistortionToneConfigureFrequency.vi"() -> ()  [unwired: 10 in, 2 out]
  n307 = call <instrlib>:"SAHarmonicDistortionToneBandwidthConfigureResolutionAutoEnabled.vi"() -> ()  [unwired: 10 in, 2 out]
  n308 = call <instrlib>:"SAHarmonicDistortionTracesInitiate.vi"() -> ()  [unwired: 10 in, 2 out]
  n309 = call <instrlib>:"SAPowerStatisticsConfigureNoPreset.vi"() -> ()  [unwired: 10 in, 2 out]
  n310 = call <instrlib>:"SystemDisableLocalControls.vi"() -> ()  [unwired: 10 in, 2 out]
  n311 = call <instrlib>:"Write Bytes.vi"() -> ()  [unwired: 10 in, 2 out]
  n312 = call <instrlib>:"Configure No Preset.vi"() -> ()  [unwired: 10 in, 2 out]
  n313 = call <instrlib>:"Configure Channel Spacing.vi"() -> ()  [unwired: 8 in, 3 out]
  n314 = call <instrlib>:"SAACPOffsetListConfigureEnabled.vi"() -> ()  [unwired: 10 in, 2 out]
  n315 = call <instrlib>:"Query Relative Limit Carrier.vi"() -> ()  [unwired: 8 in, 4 out]
  n316 = call <instrlib>:"Configure Resolution.vi"() -> ()  [unwired: 10 in, 2 out]
  n317 = call <instrlib>:"Query Video Auto Enabled.vi"() -> ()  [unwired: 8 in, 4 out]
  n318 = call <instrlib>:"SAACPOffsetListFilterConfigureEnabled.vi"() -> ()  [unwired: 10 in, 2 out]
  n319 = call <instrlib>:"SABurstPowerConfigureNoPreset.vi"() -> ()  [unwired: 10 in, 2 out]
  n320 = call <instrlib>:"SABurstPowerTracesInitiate.vi"() -> ()  [unwired: 10 in, 2 out]
  n321 = call <instrlib>:"SAChannelPowerConfigureNoPreset.vi"() -> ()  [unwired: 10 in, 2 out]
  n322 = call <instrlib>:"SAChannelPowerFrequencyLastSpan.vi"() -> ()  [unwired: 10 in, 2 out]
  n323 = call <instrlib>:"SAChannelPowerMarkerQuery.vi"() -> ()  [unwired: 8 in, 4 out]
  n324 = call <instrlib>:"SAOccupiedBandwidthConfigureNoPreset.vi"() -> ()  [unwired: 10 in, 2 out]
  n325 = call <instrlib>:"SAOccupiedBandwidthFrequencyLastSpan.vi"() -> ()  [unwired: 10 in, 2 out]
  n326 = call <instrlib>:"SAOccupiedBandwidthMarkerQuery.vi"() -> ()  [unwired: 8 in, 4 out]
  n327 = call <instrlib>:"SAOccupiedBandwidthTracesInitiate.vi"() -> ()  [unwired: 10 in, 2 out]
  n328 = call <instrlib>:"SAPowerStatisticsMarkerDisableAll.vi"() -> ()  [unwired: 10 in, 2 out]
  n329 = call <instrlib>:"SASEMaskConfigureNoPreset.vi"() -> ()  [unwired: 10 in, 2 out]
  n330 = call <instrlib>:"SASEMaskMarkerQuery.vi"() -> ()  [unwired: 8 in, 4 out]
  n331 = call <instrlib>:"Configure Relative Attenuation.vi"() -> ()  [unwired: 10 in, 2 out]
  n332 = call <instrlib>:"Configure Ratio.vi"() -> ()  [unwired: 10 in, 2 out]
  n333 = call <instrlib>:"SASEMaskOffsetListBandwidthQueryVideoAutoEnabled.vi"() -> ()  [unwired: 8 in, 4 out]
  n334 = call <instrlib>:"SASEMaskOffsetListStartConfigureFrequency.vi"() -> ()  [unwired: 10 in, 2 out]
  n335 = call <instrlib>:"Configure Absolute Amplitude Limit Couple Enabled.vi"() -> ()  [unwired: 10 in, 2 out]
  n336 = call <instrlib>:"SASEMaskTracesInitiate.vi"() -> ()  [unwired: 10 in, 2 out]
  n337 = call <instrlib>:"SASpuriousEmissionsConfigureIFGainAutoEnabled.vi"() -> ()  [unwired: 10 in, 2 out]
  n338 = call <instrlib>:"SASpuriousEmissionsMarkerDisableAll.vi"() -> ()  [unwired: 10 in, 2 out]
  n339 = call <instrlib>:"SASpuriousEmissionsRangeTableConfigureAttenuationAutoEnabled.vi"() -> ()  [unwired: 10 in, 2 out]
  n340 = call <instrlib>:"Query Attenuation Auto Enabled.vi"() -> ()  [unwired: 8 in, 4 out]
  n341 = call <instrlib>:"SASpuriousEmissionsRangeTableBandwidthConfigureResolutionAutoEnabled.vi"() -> ()  [unwired: 10 in, 2 out]
  n342 = call <instrlib>:"SASpuriousEmissionsRangeTableStartConfigureFrequency.vi"() -> ()  [unwired: 10 in, 2 out]
  n343 = call <instrlib>:"SASpuriousEmissionsRangeTableStopConfigureAbsoluteAmplitudeLimitAutoEnabled.vi"() -> ()  [unwired: 10 in, 2 out]
  n344 = call <instrlib>:"SASpuriousEmissionsTracesInitiate.vi"() -> ()  [unwired: 10 in, 2 out]
  n345 = call <instrlib>:"SASweptSAsConfigureNoPreset.vi"() -> ()  [unwired: 10 in, 2 out]
  n346 = call <instrlib>:"SAThirdOrderInterceptConfigureNoPreset.vi"() -> ()  [unwired: 10 in, 2 out]
  n347 = call <instrlib>:"SAThirdOrderInterceptTracesInitiate.vi"() -> ()  [unwired: 10 in, 2 out]
  n348 = call <instrlib>:"Clear All File Header.vi"() -> ()  [unwired: 10 in, 2 out]
  n349 = call <instrlib>:"Query Step Input Trigger Type.vi"() -> ()  [unwired: 9 in, 3 out]
  n350 = call <instrlib>:"SAACPFrequencyLastSpan.vi"() -> ()  [unwired: 10 in, 2 out]
  n351 = call <instrlib>:"Disable All.vi"() -> ()  [unwired: 10 in, 2 out]
  n352 = call <instrlib>:"SAACPTracesInitiate.vi"() -> ()  [unwired: 10 in, 2 out]
  n353 = call <instrlib>:"SAPowerStatisticsTracesInitiate.vi"() -> ()  [unwired: 10 in, 2 out]
  n354 = call <instrlib>:"Query List Step Duration Type.vi"() -> ()  [unwired: 9 in, 3 out]
  n355 = call <instrlib>:"Clear Average.vi"() -> ()  [unwired: 10 in, 2 out]
  n356 = call <instrlib>:"Query Modulation Format Test Pattern.vi"() -> ()  [unwired: 8 in, 4 out]
  n357 = call <instrlib>:"Clear List.vi"() -> ()  [unwired: 10 in, 2 out]
  n358 = call <instrlib>:"Get Line Enabled.vi"() -> ()  [unwired: 9 in, 3 out]
  n359 = call <instrlib>:"SAChannelPowerTracesInitiateSignal.vi"() -> ()  [unwired: 10 in, 2 out]
  n360 = call <instrlib>:"Get Register.vi"() -> ()  [unwired: 9 in, 3 out]
  n361 = call <instrlib>:"Set Detector Trace.vi"() -> ()  [unwired: 10 in, 2 out]
  n362 = call <instrlib>:"SAHarmonicDistortionToneBandwidthConfigureVideo.vi"() -> ()  [unwired: 10 in, 2 out]
  n363 = call <instrlib>:"Initiate.vi"() -> ()  [unwired: 10 in, 2 out]
  n364 = call <instrlib>:"Exchange Traces.vi"() -> ()  [unwired: 10 in, 2 out]
  n365 = call <instrlib>:"SABurstPowerMarkerQuery.vi"() -> ()  [unwired: 8 in, 4 out]
  n366 = call <instrlib>:"Configure Sweep Time.vi"() -> ()  [unwired: 10 in, 2 out]
  n367 = call <instrlib>:"SAHarmonicDistortionRangeTableBandwidthConfigureVideo.vi"() -> ()  [unwired: 10 in, 2 out]
  n368 = call <instrlib>:"SAHarmonicDistortionToneConfigureSpan.vi"() -> ()  [unwired: 10 in, 2 out]
  n369 = call <instrlib>:"SAPowerStatisticsDisplayStoreReferenceTrace.vi"() -> ()  [unwired: 10 in, 2 out]
  n370 = call <instrlib>:"SystemEnableLocalControls.vi"() -> ()  [unwired: 10 in, 2 out]
  n371 = call <instrlib>:"Write String.vi"() -> ()  [unwired: 10 in, 2 out]
  n372 = call <instrlib>:"Configure Coupling Enabled.vi"() -> ()  [unwired: 8 in, 3 out]
  n373 = call <instrlib>:"Configure Frequency.vi"() -> ()  [unwired: 10 in, 2 out]
  n374 = call <instrlib>:"Query Relative Limit PSD.vi"() -> ()  [unwired: 8 in, 4 out]
  n375 = call <instrlib>:"Configure Resolution Auto Enabled.vi"() -> ()  [unwired: 10 in, 2 out]
  n376 = call <instrlib>:"SABurstPowerTracesInitiateSignal.vi"() -> ()  [unwired: 10 in, 2 out]
  n377 = call <instrlib>:"SAChannelPowerMarkerSearch.vi"() -> ()  [unwired: 10 in, 2 out]
  n378 = call <instrlib>:"SAHarmonicDistortionTracesInitiateSignal.vi"() -> ()  [unwired: 10 in, 2 out]
  n379 = call <instrlib>:"SAOccupiedBandwidthMarkerSearch.vi"() -> ()  [unwired: 10 in, 2 out]
  n380 = call <instrlib>:"SAOccupiedBandwidthTracesInitiateSignal.vi"() -> ()  [unwired: 10 in, 2 out]
  n381 = call <instrlib>:"SAPowerStatisticsMarkerQuery.vi"() -> ()  [unwired: 8 in, 4 out]
  n382 = call <instrlib>:"SASEMaskOffsetListConfigureSidebandSelection.vi"() -> ()  [unwired: 10 in, 2 out]
  n383 = call <instrlib>:"Configure Ratio Auto Enabled.vi"() -> ()  [unwired: 10 in, 2 out]
  n384 = call <instrlib>:"Configure Relative Amplitude Limit.vi"() -> ()  [unwired: 10 in, 2 out]
  n385 = call <instrlib>:"SASEMaskOffsetListStopConfigureFrequency.vi"() -> ()  [unwired: 10 in, 2 out]
  n386 = call <instrlib>:"SASEMaskTracesInitiateSignal.vi"() -> ()  [unwired: 10 in, 2 out]
  n387 = call <instrlib>:"SASpuriousEmissionsConfigureIFGainState.vi"() -> ()  [unwired: 10 in, 2 out]
  n388 = call <instrlib>:"SASpuriousEmissionsMarkerQuery.vi"() -> ()  [unwired: 8 in, 4 out]
  n389 = call <instrlib>:"SASpuriousEmissionsRangeTableConfigureDetector1.vi"() -> ()  [unwired: 10 in, 2 out]
  n390 = call <instrlib>:"SASpuriousEmissionsRangeTableQueryDetector1.vi"() -> ()  [unwired: 8 in, 4 out]
  n391 = call <instrlib>:"SASpuriousEmissionsRangeTableBandwidthConfigureShape.vi"() -> ()  [unwired: 10 in, 2 out]
  n392 = call <instrlib>:"SASpuriousEmissionsRangeTableStartQueryAbsoluteAmplitudeLimit.vi"() -> ()  [unwired: 8 in, 4 out]
  n393 = call <instrlib>:"SASpuriousEmissionsRangeTableStopConfigureFrequency.vi"() -> ()  [unwired: 10 in, 2 out]
  n394 = call <instrlib>:"SASpuriousEmissionsTracesInitiateSignal.vi"() -> ()  [unwired: 10 in, 2 out]
  n395 = call <instrlib>:"SASweptSAsInitiate.vi"() -> ()  [unwired: 10 in, 2 out]
  n396 = call <instrlib>:"SAThirdOrderInterceptAutoTune.vi"() -> ()  [unwired: 10 in, 2 out]
  n397 = call <instrlib>:"SAThirdOrderInterceptTracesInitiateSignal.vi"() -> ()  [unwired: 10 in, 2 out]
  n398 = call <instrlib>:"SS Digital Modulation Arb Delete.vi"() -> ()  [unwired: 10 in, 2 out]
  n399 = call <instrlib>:"Query.vi"() -> ()  [unwired: 8 in, 4 out]
  n400 = call <instrlib>:"SAACPOffsetListFilterQueryAlpha.vi"() -> ()  [unwired: 8 in, 4 out]
  n401 = call <instrlib>:"SAACPTracesInitiateSignal.vi"() -> ()  [unwired: 10 in, 2 out]
  n402 = call <instrlib>:"SAPowerStatisticsTracesInitiateSignal.vi"() -> ()  [unwired: 10 in, 2 out]
  n403 = call <instrlib>:"Query List Step Frequency.vi"() -> ()  [unwired: 9 in, 3 out]
  n404 = call <instrlib>:"TracesInitiateSignal.vi"() -> ()  [unwired: 10 in, 2 out]
  n405 = call <instrlib>:"Is Armed.vi"() -> ()  [unwired: 9 in, 3 out]
  n406 = call <instrlib>:"Get Line.vi"() -> ()  [unwired: 9 in, 3 out]
  n407 = call <instrlib>:"Fetch Channel Density.vi"() -> ()  [unwired: 9 in, 3 out]
  n408 = call <instrlib>:"StatusPreset.vi"() -> ()  [unwired: 10 in, 2 out]
  n409 = call <instrlib>:"Set Detector Trace Auto Enabled.vi"() -> ()  [unwired: 10 in, 2 out]
  n410 = call <instrlib>:"Send Software Trigger.vi"() -> ()  [unwired: 10 in, 2 out]
  n411 = call <instrlib>:"Subtract Traces.vi"() -> ()  [unwired: 10 in, 2 out]
  n412 = call <instrlib>:"SABurstPowerMarkerSearch.vi"() -> ()  [unwired: 10 in, 2 out]
  n413 = call <instrlib>:"Configure Sweep Time Auto Enabled.vi"() -> ()  [unwired: 10 in, 2 out]
  n414 = call <instrlib>:"SAHarmonicDistortionToneBandwidthConfigureVideoAutoEnabled.vi"() -> ()  [unwired: 10 in, 2 out]
  n415 = call <instrlib>:"SASEMaskOffsetListConfigureSweepTime.vi"() -> ()  [unwired: 10 in, 2 out]
  n416 = call <instrlib>:"SASEMaskOffsetListBandwidthConfigureResolution.vi"() -> ()  [unwired: 10 in, 2 out]
  n417 = call <instrlib>:"SASpuriousEmissionsConfigureNoPreset.vi"() -> ()  [unwired: 10 in, 2 out]
  n418 = call <instrlib>:"SASpuriousEmissionsMarkerSearch.vi"() -> ()  [unwired: 10 in, 2 out]
  n419 = call <instrlib>:"SASpuriousEmissionsRangeTableConfigureDetector2.vi"() -> ()  [unwired: 10 in, 2 out]
  n420 = call <instrlib>:"SASpuriousEmissionsRangeTableQueryDetector2.vi"() -> ()  [unwired: 8 in, 4 out]
  n421 = call <instrlib>:"SASpuriousEmissionsRangeTableBandwidthConfigureVideo.vi"() -> ()  [unwired: 10 in, 2 out]
  n422 = call <instrlib>:"SASpuriousEmissionsRangeTableStartQueryFrequency.vi"() -> ()  [unwired: 8 in, 4 out]
  n423 = call <instrlib>:"SASpuriousEmissionsRangeTableStopQueryAbsoluteAmplitudeLimit.vi"() -> ()  [unwired: 8 in, 4 out]
  n424 = call <instrlib>:"SystemGetScreenImage.vi"() -> ()  [unwired: 8 in, 4 out]
  n425 = call <instrlib>:"Configure Integration Bandwidth.vi"() -> ()  [unwired: 8 in, 3 out]
  n426 = call <instrlib>:"Configure Lower Limit.vi"() -> ()  [unwired: 10 in, 2 out]
  n427 = call <instrlib>:"Query Sideband Selection.vi"() -> ()  [unwired: 8 in, 4 out]
  n428 = call <instrlib>:"Configure Shape.vi"() -> ()  [unwired: 10 in, 2 out]
  n429 = call <instrlib>:"SAHarmonicDistortionRangeTableBandwidthConfigureVideoAutoEnabled.vi"() -> ()  [unwired: 10 in, 2 out]
  n430 = call <instrlib>:"SAHarmonicDistortionToneConfigureSweepTime.vi"() -> ()  [unwired: 10 in, 2 out]
  n431 = call <instrlib>:"Fetch Amplitude.vi"() -> ()  [unwired: 9 in, 3 out]
  n432 = call <instrlib>:"Fetch Occupied Band Width.vi"() -> ()  [unwired: 9 in, 3 out]
  n433 = call <instrlib>:"Query Absolute Amplitude Limit.vi"() -> ()  [unwired: 8 in, 4 out]
  n434 = call <instrlib>:"SASEMaskOffsetListStopConfigureRelativeAmplitudeLimit.vi"() -> ()  [unwired: 10 in, 2 out]
  n435 = call <instrlib>:"SS Digital Modulation Arb Delete All.vi"() -> ()  [unwired: 10 in, 2 out]
  n436 = call <instrlib>:"User Preset All Modes.vi"() -> ()  [unwired: 10 in, 2 out]
  n437 = call <instrlib>:"Search.vi"() -> ()  [unwired: 10 in, 2 out]
  n438 = call <instrlib>:"SAACPOffsetListFilterQueryEnabled.vi"() -> ()  [unwired: 8 in, 4 out]
  n439 = call <instrlib>:"SAPowerStatisticsTracesStoreAsReference.vi"() -> ()  [unwired: 10 in, 2 out]
  n440 = call <instrlib>:"Read Intercept Power.vi"() -> ()  [unwired: 9 in, 3 out]
  n441 = call <instrlib>:"Query List Step Radio Band Link.vi"() -> ()  [unwired: 9 in, 3 out]
  n442 = call <instrlib>:"SS List Sequencer Initiate.vi"() -> ()  [unwired: 10 in, 2 out]
  n443 = call <instrlib>:"Get Time Line Enabled.vi"() -> ()  [unwired: 9 in, 3 out]
  n444 = call <instrlib>:"Fetch Channel Power.vi"() -> ()  [unwired: 9 in, 3 out]
  n445 = call <instrlib>:"StatusSetRegister.vi"() -> ()  [unwired: 10 in, 2 out]
  n446 = call <instrlib>:"Trigger Frame Reset.vi"() -> ()  [unwired: 10 in, 2 out]
  n447 = call <instrlib>:"SASEMaskOffsetListConfigureSweepTimeAutoEnabled.vi"() -> ()  [unwired: 10 in, 2 out]
  n448 = call <instrlib>:"SASEMaskOffsetListBandwidthConfigureResolutionAutoEnabled.vi"() -> ()  [unwired: 10 in, 2 out]
  n449 = call <instrlib>:"Query IF Gain Auto Enabled.vi"() -> ()  [unwired: 8 in, 4 out]
  n450 = call <instrlib>:"SASpuriousEmissionsRangeTableConfigureEnabled.vi"() -> ()  [unwired: 10 in, 2 out]
  n451 = call <instrlib>:"SASpuriousEmissionsRangeTableQueryEnabled.vi"() -> ()  [unwired: 8 in, 4 out]
  n452 = call <instrlib>:"SASpuriousEmissionsRangeTableBandwidthConfigureVideoAutoEnabled.vi"() -> ()  [unwired: 10 in, 2 out]
  n453 = call <instrlib>:"SASpuriousEmissionsRangeTableStopQueryAbsoluteAmplitudeLimitAutoEnabled.vi"() -> ()  [unwired: 8 in, 4 out]
  n454 = call <instrlib>:"Query List Step Radio Band.vi"() -> ()  [unwired: 9 in, 3 out]
  n455 = call <instrlib>:"SystemGetState.vi"() -> ()  [unwired: 8 in, 4 out]
  n456 = call <instrlib>:"Configure Method.vi"() -> ()  [unwired: 8 in, 3 out]
  n457 = call <instrlib>:"Configure Relative Limit Carrier.vi"() -> ()  [unwired: 10 in, 2 out]
  n458 = call <instrlib>:"Query Test.vi"() -> ()  [unwired: 8 in, 4 out]
  n459 = call <instrlib>:"Configure Type.vi"() -> ()  [unwired: 10 in, 2 out]
  n460 = call <instrlib>:"Configure Tone Enabled.vi"() -> ()  [unwired: 10 in, 2 out]
  n461 = call <instrlib>:"SAHarmonicDistortionRangeTableBandwidthQueryResolution.vi"() -> ()  [unwired: 8 in, 4 out]
  n462 = call <instrlib>:"SAHarmonicDistortionToneConfigureSweepTimeAutoEnabled.vi"() -> ()  [unwired: 10 in, 2 out]
  n463 = call <instrlib>:"SAHarmonicDistortionToneBandwidthQueryResolution.vi"() -> ()  [unwired: 9 in, 3 out]
  n464 = call <instrlib>:"Fetch Frequency.vi"() -> ()  [unwired: 9 in, 3 out]
  n465 = call <instrlib>:"Fetch Transmit Frequency Error.vi"() -> ()  [unwired: 9 in, 3 out]
  n466 = call <instrlib>:"SASEMaskOffsetListStartQueryFrequency.vi"() -> ()  [unwired: 8 in, 4 out]
  n467 = call <instrlib>:"Configure Relative Amplitude Limit Auto Enabled.vi"() -> ()  [unwired: 10 in, 2 out]
  n468 = call <instrlib>:"Get Header Description.vi"() -> ()  [unwired: 9 in, 3 out]
  n469 = call <instrlib>:"Mode Preset.vi"() -> ()  [unwired: 10 in, 2 out]
  n470 = call <instrlib>:"Fetch Intercept Power.vi"() -> ()  [unwired: 9 in, 3 out]
  n471 = call <instrlib>:"Get Time Line.vi"() -> ()  [unwired: 9 in, 3 out]
  n472 = call <instrlib>:"Read Channel Desnsity.vi"() -> ()  [unwired: 9 in, 3 out]
  n473 = call <instrlib>:"Get Status Register.vi"() -> ()  [unwired: 9 in, 3 out]
  n474 = call <instrlib>:"SASEMaskOffsetListConfigureTest.vi"() -> ()  [unwired: 10 in, 2 out]
  n475 = call <instrlib>:"SASEMaskOffsetListBandwidthConfigureVideo.vi"() -> ()  [unwired: 10 in, 2 out]
  n476 = call <instrlib>:"Query IF Gain State.vi"() -> ()  [unwired: 8 in, 4 out]
  n477 = call <instrlib>:"SASpuriousEmissionsRangeTableConfigurePeakExcursion.vi"() -> ()  [unwired: 10 in, 2 out]
  n478 = call <instrlib>:"Query Peak Excursion.vi"() -> ()  [unwired: 8 in, 4 out]
  n479 = call <instrlib>:"SASpuriousEmissionsRangeTableBandwidthQueryResolution.vi"() -> ()  [unwired: 8 in, 4 out]
  n480 = call <instrlib>:"SASpuriousEmissionsRangeTableStopQueryFrequency.vi"() -> ()  [unwired: 8 in, 4 out]
  n481 = call <instrlib>:"Query List Step Transition Time.vi"() -> ()  [unwired: 9 in, 3 out]
  n482 = call <instrlib>:"Auto Fill.vi"() -> ()  [unwired: 10 in, 2 out]
  n483 = call <instrlib>:"SAHarmonicDistortionRangeTableBandwidthQueryResolutionAutoEnabled.vi"() -> ()  [unwired: 8 in, 4 out]
  n484 = call <instrlib>:"SAHarmonicDistortionToneQueryEnabled.vi"() -> ()  [unwired: 9 in, 3 out]
  n485 = call <instrlib>:"SAHarmonicDistortionToneBandwidthQueryResolutionAutoEnabled.vi"() -> ()  [unwired: 9 in, 3 out]
  n486 = call <instrlib>:"Get Marker Polarity.vi"() -> ()  [unwired: 9 in, 3 out]
  n487 = call <instrlib>:"SystemPutState.vi"() -> ()  [unwired: 10 in, 2 out]
  n488 = call <instrlib>:"Configure Power Present.vi"() -> ()  [unwired: 8 in, 3 out]
  n489 = call <instrlib>:"Configure Relative Limit PSD.vi"() -> ()  [unwired: 10 in, 2 out]
  n490 = call <instrlib>:"Query Upper Limit.vi"() -> ()  [unwired: 8 in, 4 out]
  n491 = call <instrlib>:"Configure Video.vi"() -> ()  [unwired: 10 in, 2 out]
  n492 = call <instrlib>:"Fetch Fundamental Frequency.vi"() -> ()  [unwired: 9 in, 3 out]
  n493 = call <instrlib>:"Query Relative Amplitude Limit.vi"() -> ()  [unwired: 8 in, 4 out]
  n494 = call <instrlib>:"SASEMaskOffsetListStopQueryAbsoluteAmplitudeLimit.vi"() -> ()  [unwired: 8 in, 4 out]
  n495 = call <instrlib>:"Fetch XDB.vi"() -> ()  [unwired: 9 in, 3 out]
  n496 = call <instrlib>:"Set Frequency Line Enabled.vi"() -> ()  [unwired: 10 in, 2 out]
  n497 = call <instrlib>:"Read Channel Power.vi"() -> ()  [unwired: 9 in, 3 out]
  n498 = call <instrlib>:"Set Status Register.vi"() -> ()  [unwired: 10 in, 2 out]
  n499 = call <instrlib>:"Query List Step Waveform.vi"() -> ()  [unwired: 9 in, 3 out]
  n500 = call <instrlib>:"SASEMaskOffsetListQueryEnabled.vi"() -> ()  [unwired: 8 in, 4 out]
  n501 = call <instrlib>:"SASEMaskOffsetListBandwidthConfigureVideoAutoEnabled.vi"() -> ()  [unwired: 10 in, 2 out]
  n502 = call <instrlib>:"SASpuriousEmissionsRangeTableConfigurePeakThreshold.vi"() -> ()  [unwired: 10 in, 2 out]
  n503 = call <instrlib>:"Query Peak Threshold.vi"() -> ()  [unwired: 8 in, 4 out]
  n504 = call <instrlib>:"SASpuriousEmissionsRangeTableBandwidthQueryResolutionAutoEnabled.vi"() -> ()  [unwired: 8 in, 4 out]
  n505 = call <instrlib>:"SAHarmonicDistortionRangeTableQueryFrequency.vi"() -> ()  [unwired: 8 in, 4 out]
  n506 = call <instrlib>:"SAHarmonicDistortionRangeTableBandwidthQueryVideo.vi"() -> ()  [unwired: 8 in, 4 out]
  n507 = call <instrlib>:"SAHarmonicDistortionToneQueryFrequency.vi"() -> ()  [unwired: 9 in, 3 out]
  n508 = call <instrlib>:"SAHarmonicDistortionToneBandwidthQueryVideo.vi"() -> ()  [unwired: 9 in, 3 out]
  n509 = call <instrlib>:"Query Carrier Method.vi"() -> ()  [unwired: 8 in, 4 out]
  n510 = call <instrlib>:"Fetch Harmonic Distortion.vi"() -> ()  [unwired: 9 in, 3 out]
  n511 = call <instrlib>:"Query Absolute Amplitude Limit Couple Enabled.vi"() -> ()  [unwired: 8 in, 4 out]
  n512 = call <instrlib>:"Initiate Trigger.vi"() -> ()  [unwired: 10 in, 2 out]
  n513 = call <instrlib>:"SystemReadBytes.vi"() -> ()  [unwired: 8 in, 4 out]
  n514 = call <instrlib>:"Configure Sideband Selection.vi"() -> ()  [unwired: 10 in, 2 out]
  n515 = call <instrlib>:"Configure Video Auto Enabled.vi"() -> ()  [unwired: 10 in, 2 out]
  n516 = call <instrlib>:"Read Occupied Bandwidth.vi"() -> ()  [unwired: 9 in, 3 out]
  n517 = call <instrlib>:"Set Frequency Line.vi"() -> ()  [unwired: 10 in, 2 out]
  n518 = call <instrlib>:"SS List Sequencer Setup Trigger Initiate.vi"() -> ()  [unwired: 10 in, 2 out]
  n519 = call <instrlib>:"Query Span.vi"() -> ()  [unwired: 8 in, 4 out]
  n520 = call <instrlib>:"SAHarmonicDistortionRangeTableBandwidthQueryVideoAutoEnabled.vi"() -> ()  [unwired: 8 in, 4 out]
  n521 = call <instrlib>:"SAHarmonicDistortionToneQuerySpan.vi"() -> ()  [unwired: 9 in, 3 out]
  n522 = call <instrlib>:"SAHarmonicDistortionToneBandwidthQueryVideoAutoEnabled.vi"() -> ()  [unwired: 9 in, 3 out]
  n523 = call <instrlib>:"Query Relative Attenuation.vi"() -> ()  [unwired: 8 in, 4 out]
  n524 = call <instrlib>:"Query Measurement Multiplier.vi"() -> ()  [unwired: 8 in, 4 out]
  n525 = call <instrlib>:"Query Channel Spacing.vi"() -> ()  [unwired: 8 in, 4 out]
  n526 = call <instrlib>:"Read Amplitude.vi"() -> ()  [unwired: 9 in, 3 out]
  n527 = call <instrlib>:"Configure Test.vi"() -> ()  [unwired: 10 in, 2 out]
  n528 = call <instrlib>:"Query Reference.vi"() -> ()  [unwired: 8 in, 4 out]
  n529 = call <instrlib>:"SASEMaskOffsetListStopQueryFrequency.vi"() -> ()  [unwired: 8 in, 4 out]
  n530 = call <instrlib>:"Query Catalog.vi"() -> ()  [unwired: 6 in, 6 out]
  n531 = call <instrlib>:"SystemReadString.vi"() -> ()  [unwired: 9 in, 3 out]
  n532 = call <instrlib>:"SASpuriousEmissionsRangeTableConfigureSweepPoints.vi"() -> ()  [unwired: 10 in, 2 out]
  n533 = call <instrlib>:"Query Sweep Points.vi"() -> ()  [unwired: 8 in, 4 out]
  n534 = call <instrlib>:"SASpuriousEmissionsRangeTableBandwidthQueryShape.vi"() -> ()  [unwired: 8 in, 4 out]
  n535 = call <instrlib>:"Read Transmit Frequency Error.vi"() -> ()  [unwired: 9 in, 3 out]
  n536 = call <instrlib>:"Set Line Enabled.vi"() -> ()  [unwired: 10 in, 2 out]
  n537 = call <instrlib>:"SAHarmonicDistortionToneQuerySweepTime.vi"() -> ()  [unwired: 9 in, 3 out]
  n538 = call <instrlib>:"SASEMaskOffsetListQuerySidebandSelection.vi"() -> ()  [unwired: 8 in, 4 out]
  n539 = call <instrlib>:"Query Ratio.vi"() -> ()  [unwired: 8 in, 4 out]
  n540 = call <instrlib>:"Query Coupling Enabled.vi"() -> ()  [unwired: 8 in, 4 out]
  n541 = call <instrlib>:"Query Sweep Time.vi"() -> ()  [unwired: 8 in, 4 out]
  n542 = call <instrlib>:"Read Frequency.vi"() -> ()  [unwired: 9 in, 3 out]
  n543 = call <instrlib>:"Query Locked Waveform List.vi"() -> ()  [unwired: 9 in, 3 out]
  n544 = call <instrlib>:"Configure Upper Limit.vi"() -> ()  [unwired: 10 in, 2 out]
  n545 = call <instrlib>:"Query Resolution.vi"() -> ()  [unwired: 8 in, 4 out]
  n546 = call <instrlib>:"SASEMaskOffsetListStopQueryRelativeAmplitudeLimit.vi"() -> ()  [unwired: 8 in, 4 out]
  n547 = call <instrlib>:"SystemRecallState.vi"() -> ()  [unwired: 10 in, 2 out]
  n548 = call <instrlib>:"SASpuriousEmissionsRangeTableConfigureSweepPointsAutoEnabled.vi"() -> ()  [unwired: 10 in, 2 out]
  n549 = call <instrlib>:"Query Sweep Points Auto Enabled.vi"() -> ()  [unwired: 8 in, 4 out]
  n550 = call <instrlib>:"SASpuriousEmissionsRangeTableBandwidthQueryVideo.vi"() -> ()  [unwired: 8 in, 4 out]
  n551 = call <instrlib>:"Read XDB.vi"() -> ()  [unwired: 9 in, 3 out]
  n552 = call <instrlib>:"Set Line.vi"() -> ()  [unwired: 10 in, 2 out]
  n553 = call <instrlib>:"SAHarmonicDistortionToneQuerySweepTimeAutoEnabled.vi"() -> ()  [unwired: 9 in, 3 out]
  n554 = call <instrlib>:"Query Sweep Time Auto Enabled.vi"() -> ()  [unwired: 8 in, 4 out]
  n555 = call <instrlib>:"Read Fundamental Frequency.vi"() -> ()  [unwired: 9 in, 3 out]
  n556 = call <instrlib>:"SASEMaskOffsetListQuerySweepTime.vi"() -> ()  [unwired: 8 in, 4 out]
  n557 = call <instrlib>:"Query Ratio Auto Enabled.vi"() -> ()  [unwired: 8 in, 4 out]
  n558 = call <instrlib>:"Query Integration Bandwidth.vi"() -> ()  [unwired: 8 in, 4 out]
  n559 = call <instrlib>:"Save Header.vi"() -> ()  [unwired: 10 in, 2 out]
  n560 = call <instrlib>:"Query Absolute Limit.vi"() -> ()  [unwired: 8 in, 4 out]
  n561 = call <instrlib>:"Query Resolution Auto Enabled.vi"() -> ()  [unwired: 8 in, 4 out]
  n562 = call <instrlib>:"Query Relative Amplitude Limit Auto Enabled.vi"() -> ()  [unwired: 8 in, 4 out]
  n563 = call <instrlib>:"SystemSaveState.vi"() -> ()  [unwired: 10 in, 2 out]
  n564 = call <instrlib>:"SASpuriousEmissionsRangeTableConfigureSweepTime.vi"() -> ()  [unwired: 10 in, 2 out]
  n565 = call <instrlib>:"SASpuriousEmissionsRangeTableQuerySweepTime.vi"() -> ()  [unwired: 8 in, 4 out]
  n566 = call <instrlib>:"SASpuriousEmissionsRangeTableBandwidthQueryVideoAutoEnabled.vi"() -> ()  [unwired: 8 in, 4 out]
  n567 = call <instrlib>:"Set Time Line Enabled.vi"() -> ()  [unwired: 10 in, 2 out]
  n568 = call <instrlib>:"Query Tone Enabled.vi"() -> ()  [unwired: 8 in, 4 out]
  n569 = call <instrlib>:"Read Harmonic Distortion.vi"() -> ()  [unwired: 9 in, 3 out]
  n570 = call <instrlib>:"SASEMaskOffsetListQuerySweepTimeAutoEnabled.vi"() -> ()  [unwired: 8 in, 4 out]
  n571 = call <instrlib>:"SASEMaskOffsetListBandwidthQueryResolution.vi"() -> ()  [unwired: 8 in, 4 out]
  n572 = call <instrlib>:"Query Method.vi"() -> ()  [unwired: 8 in, 4 out]
  n573 = call <instrlib>:"Set Marker Polarity.vi"() -> ()  [unwired: 10 in, 2 out]
  n574 = call <instrlib>:"SAACPOffsetListQueryEnabled.vi"() -> ()  [unwired: 8 in, 4 out]
  n575 = call <instrlib>:"Query Shape.vi"() -> ()  [unwired: 8 in, 4 out]
  n576 = call <instrlib>:"viRead.vi"() -> ()  [unwired: 8 in, 4 out]
  n577 = call <instrlib>:"SASpuriousEmissionsRangeTableConfigureSweepTimeAutoEnabled.vi"() -> ()  [unwired: 10 in, 2 out]
  n578 = call <instrlib>:"SASpuriousEmissionsRangeTableQuerySweepTimeAutoEnabled.vi"() -> ()  [unwired: 8 in, 4 out]
  n579 = call <instrlib>:"Set Time Line.vi"() -> ()  [unwired: 10 in, 2 out]
  n580 = call <instrlib>:"SASEMaskOffsetListQueryTest.vi"() -> ()  [unwired: 8 in, 4 out]
  n581 = call <instrlib>:"SASEMaskOffsetListBandwidthQueryResolutionAutoEnabled.vi"() -> ()  [unwired: 8 in, 4 out]
  n582 = call <instrlib>:"Query Power Present.vi"() -> ()  [unwired: 8 in, 4 out]
  n583 = call <instrlib>:"Query Frequency.vi"() -> ()  [unwired: 8 in, 4 out]
  n584 = call <instrlib>:"Query Type.vi"() -> ()  [unwired: 8 in, 4 out]
  n585 = call <instrlib>:"viWrite.vi"() -> ()  [unwired: 9 in, 3 out]
  n586 = call <instrlib>:"SASpuriousEmissionsRangeTableConfigureSweepTimeAutoRules.vi"() -> ()  [unwired: 10 in, 2 out]
  n587 = call <instrlib>:"SASpuriousEmissionsRangeTableQuerySweepTimeAutoRules.vi"() -> ()  [unwired: 8 in, 4 out]
  n588 = call <instrlib>:"SAACPTraceFetch.vi"() -> ()  [unwired: 8 in, 4 out]
  n589 = call <instrlib>:"Fetch Y Trace.vi"() -> ()  [unwired: 8 in, 4 out]
  n590 = call <instrlib>:"SABurstPowerTraceFetch.vi"() -> ()  [unwired: 8 in, 4 out]
  n591 = call <instrlib>:"SAChannelPowerTraceFetch.vi"() -> ()  [unwired: 8 in, 4 out]
  n592 = call <instrlib>:"SAHarmonicDistortionTraceFetch.vi"() -> ()  [unwired: 8 in, 4 out]
  n593 = call <instrlib>:"SAListSweepFetch.vi"() -> ()  [unwired: 8 in, 4 out]
  n594 = call <instrlib>:"SAOccupiedBandwidthTraceFetch.vi"() -> ()  [unwired: 8 in, 4 out]
  n595 = call <instrlib>:"SAPowerStatisticsTraceFetch.vi"() -> ()  [unwired: 8 in, 4 out]
  n596 = call <instrlib>:"SASEMaskTraceFetch.vi"() -> ()  [unwired: 8 in, 4 out]
  n597 = call <instrlib>:"SASpuriousEmissionsTraceFetch.vi"() -> ()  [unwired: 8 in, 4 out]
  n598 = call <instrlib>:"SASweptSAFetch.vi"() -> ()  [unwired: 8 in, 4 out]
  n599 = call <instrlib>:"SAThirdOrderInterceptTraceFetch.vi"() -> ()  [unwired: 8 in, 4 out]
  n600 = call <instrlib>:"Query List Duration Time.vi"() -> ()  [unwired: 8 in, 4 out]
  n601 = call <instrlib>:"TraceClear.vi"() -> ()  [unwired: 10 in, 2 out]
  n602 = call <instrlib>:"Read Y Trace.vi"() -> ()  [unwired: 8 in, 4 out]
  n603 = call <instrlib>:"SAACPTraceRead.vi"() -> ()  [unwired: 8 in, 4 out]
  n604 = call <instrlib>:"SABurstPowerTraceRead.vi"() -> ()  [unwired: 8 in, 4 out]
  n605 = call <instrlib>:"SAChannelPowerTraceRead.vi"() -> ()  [unwired: 8 in, 4 out]
  n606 = call <instrlib>:"SAHarmonicDistortionTraceRead.vi"() -> ()  [unwired: 8 in, 4 out]
  n607 = call <instrlib>:"SAListSweepMeasure.vi"() -> ()  [unwired: 8 in, 4 out]
  n608 = call <instrlib>:"SAOccupiedBandwidthTraceRead.vi"() -> ()  [unwired: 8 in, 4 out]
  n609 = call <instrlib>:"SAPowerStatisticsTraceRead.vi"() -> ()  [unwired: 8 in, 4 out]
  n610 = call <instrlib>:"SASEMaskTraceRead.vi"() -> ()  [unwired: 8 in, 4 out]
  n611 = call <instrlib>:"SASpuriousEmissionsTraceRead.vi"() -> ()  [unwired: 8 in, 4 out]
  n612 = call <instrlib>:"SASweptSAMeasure.vi"() -> ()  [unwired: 8 in, 4 out]
  n613 = call <instrlib>:"SAThirdOrderInterceptTraceRead.vi"() -> ()  [unwired: 8 in, 4 out]
  n614 = call <instrlib>:"Query List Duration Type.vi"() -> ()  [unwired: 8 in, 4 out]
  n615 = call <instrlib>:"Compress.vi"() -> ()  [unwired: 12 in, 4 out]
  n616 = call <instrlib>:"Query List Frequency.vi"() -> ()  [unwired: 8 in, 4 out]
  n617 = call <instrlib>:"SAACPTraceReadSignal.vi"() -> ()  [unwired: 12 in, 4 out]
  n618 = call <instrlib>:"SABurstPowerTraceReadSignal.vi"() -> ()  [unwired: 12 in, 4 out]
  n619 = call <instrlib>:"SAChannelPowerTraceReadSignal.vi"() -> ()  [unwired: 12 in, 4 out]
  n620 = call <instrlib>:"SAHarmonicDistortionTraceReadSignal.vi"() -> ()  [unwired: 12 in, 4 out]
  n621 = call <instrlib>:"SAListSweepRead.vi"() -> ()  [unwired: 8 in, 4 out]
  n622 = call <instrlib>:"SAOccupiedBandwidthTraceReadSignal.vi"() -> ()  [unwired: 12 in, 4 out]
  n623 = call <instrlib>:"SAPowerStatisticsTraceReadSignal.vi"() -> ()  [unwired: 12 in, 4 out]
  n624 = call <instrlib>:"SASEMaskTraceReadSignal.vi"() -> ()  [unwired: 12 in, 4 out]
  n625 = call <instrlib>:"SASpuriousEmissionsTraceReadSignal.vi"() -> ()  [unwired: 12 in, 4 out]
  n626 = call <instrlib>:"SASweptSARead.vi"() -> ()  [unwired: 8 in, 4 out]
  n627 = call <instrlib>:"SAThirdOrderInterceptTraceReadSignal.vi"() -> ()  [unwired: 12 in, 4 out]
  n628 = call <instrlib>:"Export Trace CSV.vi"() -> ()  [unwired: 10 in, 2 out]
  n629 = call <instrlib>:"Query List Power.vi"() -> ()  [unwired: 8 in, 4 out]
  n630 = call <instrlib>:"Read Frequency All.vi"() -> ()  [unwired: 8 in, 4 out]
  n631 = call <instrlib>:"FetchX.vi"() -> ()  [unwired: 8 in, 4 out]
  n632 = call <instrlib>:"Query List Radio Band Link.vi"() -> ()  [unwired: 8 in, 4 out]
  n633 = call <instrlib>:"Fetch Frequency All.vi"() -> ()  [unwired: 8 in, 4 out]
  n634 = call <instrlib>:"TraceImportTraceCSV.vi"() -> ()  [unwired: 10 in, 2 out]
  n635 = call <instrlib>:"Query List Radio Band.vi"() -> ()  [unwired: 8 in, 4 out]
  n636 = call <instrlib>:"Fetch Amplitude All.vi"() -> ()  [unwired: 8 in, 4 out]
  n637 = call <instrlib>:"Peaks.vi"() -> ()  [unwired: 12 in, 4 out]
  n638 = call <instrlib>:"Read Amplitude All.vi"() -> ()  [unwired: 8 in, 4 out]
  n639 = call <instrlib>:"Disable.vi"() -> ()  [unwired: 10 in, 2 out]
  n640 = call <instrlib>:"MemoryOperationCopy.vi"() -> ()  [unwired: 10 in, 2 out]
  n641 = call <instrlib>:"Set Storage Directory.vi"() -> ()  [unwired: 10 in, 2 out]
  n642 = call <instrlib>:"Move.vi"() -> ()  [unwired: 10 in, 2 out]
  n643 = call <instrlib>:"Remove Storage Directory.vi"() -> ()  [unwired: 10 in, 2 out]
  n644 = call <instrlib>:"Calibrate Conducted Band.vi"() -> ()  [unwired: 10 in, 2 out]
  n645 = call <instrlib>:"Query Align Radiated Band Timestamp.vi"() -> ()  [unwired: 9 in, 3 out]
  n646 = call <instrlib>:"Zoom In.vi"() -> ()  [unwired: 10 in, 2 out]
  n647 = call <instrlib>:"Calibrate.vi"() -> ()  [unwired: 10 in, 2 out]
  n648 = call <instrlib>:"Error Message.vi"() -> ()  [unwired: 9 in, 3 out]
  n649 = call <instrlib>:"Calibrate Full Band.vi"() -> ()  [unwired: 10 in, 2 out]
  n650 = call <instrlib>:"Create Storage Directory.vi"() -> ()  [unwired: 10 in, 2 out]
  n651 = call <instrlib>:"Store Correction Data To File.vi"() -> ()  [unwired: 10 in, 2 out]
  n652 = call <instrlib>:"Query Directory Catalog.vi"() -> ()  [unwired: 9 in, 3 out]
  n653 = call <instrlib>:"Store State.vi"() -> ()  [unwired: 10 in, 2 out]
  n654 = call <instrlib>:"Calibrate Expired Alignment.vi"() -> ()  [unwired: 9 in, 3 out]
  n655 = call <instrlib>:"Zoom Out.vi"() -> ()  [unwired: 10 in, 2 out]
  n656 = call <instrlib>:"Reset.vi"() -> ()  [unwired: 10 in, 2 out]
  n657 = call <instrlib>:"Calibrate Radiated Band.vi"() -> ()  [unwired: 10 in, 2 out]
  n658 = call <instrlib>:"MemoryOperationDelete.vi"() -> ()  [unwired: 10 in, 2 out]
  n659 = call <instrlib>:"Store Marker Table To File.vi"() -> ()  [unwired: 10 in, 2 out]
  n660 = call <instrlib>:"Query Storage Directory.vi"() -> ()  [unwired: 9 in, 3 out]
  n661 = call <instrlib>:"Store Trace To Register.vi"() -> ()  [unwired: 10 in, 2 out]
  n662 = call <instrlib>:"Revision Query.vi"() -> ()  [unwired: 8 in, 4 out]
  n663 = call <instrlib>:"Query Align Conducted Band Temprature.vi"() -> ()  [unwired: 9 in, 3 out]
  n664 = call <instrlib>:"Limit Data To File.vi"() -> ()  [unwired: 10 in, 2 out]
  n665 = call <instrlib>:"Store Measurement Results To File.vi"() -> ()  [unwired: 10 in, 2 out]
  n666 = call <instrlib>:"Recall State.vi"() -> ()  [unwired: 10 in, 2 out]
  n667 = call <instrlib>:"Store Trace To Trace File.vi"() -> ()  [unwired: 10 in, 2 out]
  n668 = call <instrlib>:"Query Align Conducted Band Timestamp.vi"() -> ()  [unwired: 9 in, 3 out]
  n669 = call <instrlib>:"Load Correction File Data.vi"() -> ()  [unwired: 10 in, 2 out]
  n670 = call <instrlib>:"Store Peak Table To File.vi"() -> ()  [unwired: 10 in, 2 out]
  n671 = call <instrlib>:"Recall Trace From Register.vi"() -> ()  [unwired: 10 in, 2 out]
  n672 = call <instrlib>:"Query Align Radiated Band Temprature.vi"() -> ()  [unwired: 9 in, 3 out]
  n673 = call <instrlib>:"Load Limit File Data.vi"() -> ()  [unwired: 10 in, 2 out]
  n674 = call <instrlib>:"Store Screen Image To File.vi"() -> ()  [unwired: 10 in, 2 out]
  n675 = call <instrlib>:"Recall Trace From Trace File.vi"() -> ()  [unwired: 10 in, 2 out]
  n676 = call <instrlib>:"Close.vi"() -> ()  [unwired: 11 in, 1 out]
